vi "ACQ get internal temp.vi"(4 "pomiar temp (T)":bool=TRUE, 6 "i":i32, 7 "Urządzenie":tag, 8 "error in (no error)":errorcluster, 9 "div (300)":i32=300, 11 "Tasks ref in":T1) -> (0 "error out":errorcluster, 3 "Tasks ref out":T1, 5 "DevTemp":dbl)   [LabVIEW 2014]
doc: "Odczytuje temperaturę urządzenia co zadaną liczbę iteracji (div)\nprzerywając zadania pomiarowe.\n(div 125 to ok 1 sek przy pętli ok 0,008s)"
uses:
  Kontrolki/KartaDAQ/ACQ all read tasks.ctl
  <resource>/objmgr/daqmx.rc
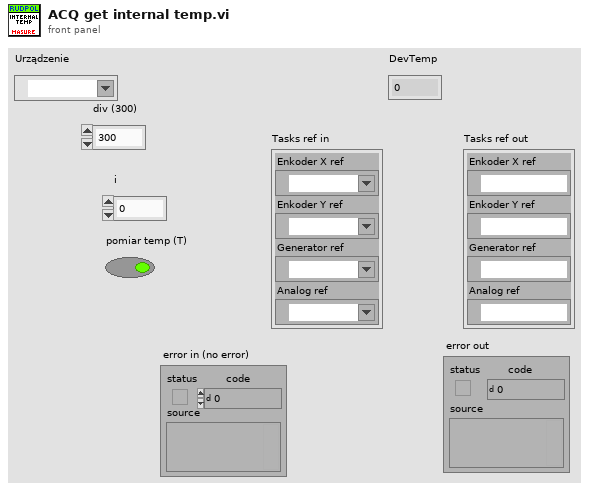
[diagram p1: front panel]
types:
  T1 = typedef "ACQ all read tasks.ctl" = cluster{"Analog ref":refnum<k21>, "Enkoder X ref":refnum<k21>, "Enkoder Y ref":refnum<k21>, "Generator ref":refnum<k21>}
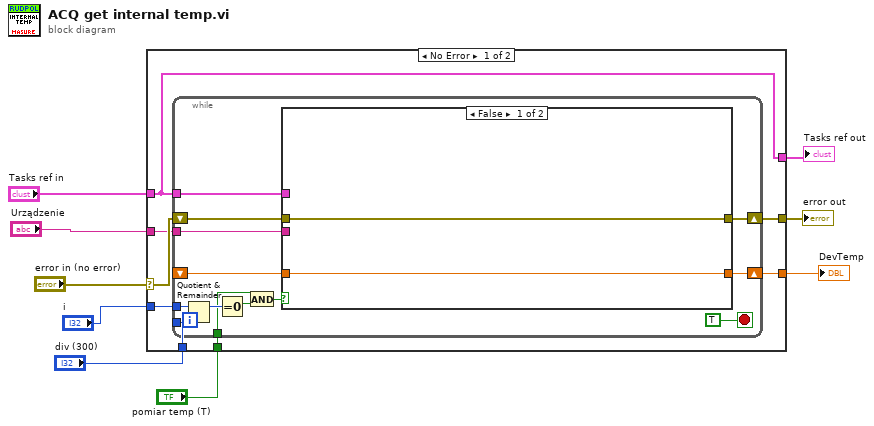
[diagram p0: block diagram]
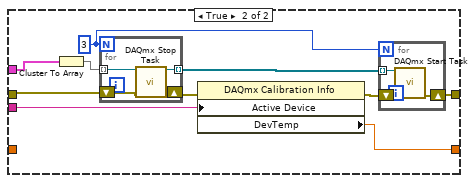
[diagram p2: hidden frame]
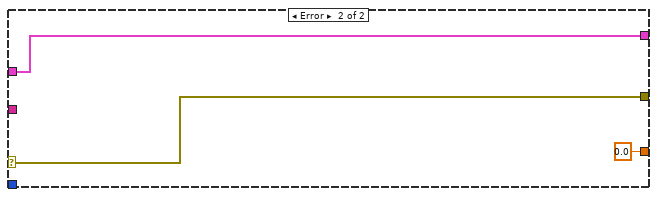
[diagram p3: hidden frame]
diagram:
  n1 = case shown="No Error" "error in (no error)" {
    selector: "error in (no error)" -> [w17 w52]
    tunnel: [w15 w52] -> w8
    tunnel: "Tasks ref in" -> [w16 w51]
    tunnel: [w16 w51] -> w6
    tunnel: "Urządzenie" -> [w14 _]
    tunnel: "i" -> [w13 _]
    tunnel: "div (300)" -> [w12 _]
    tunnel: [w11 0.0 ("DevTemp")] -> w2
    tunnel: "pomiar temp (T)" -> [w10 _]
    frame No Error {
      n2 = while {
        tunnel: w16 -> [w29]
        tunnel: w14 -> [w27]
        tunnel: w13 -> [w25]
        tunnel: w12 -> [w24]
        shift-right: [w28] -> w15
        shift-left: w17 -> [w30]
        shift-right: [w23] -> w11
        shift-left: _ -> [w21]
        tunnel: w10 -> [w18]
        stop <- TRUE stop-if-true
        n3 = Quotient & Remainder(x=w25, y=w24) -> (x-y*floor(x/y)=w26:i32)  [unwired: 1 out]
        n4 = Equal To 0?(x=w26) -> (x = 0?=w19:bool)
        n5 = And(x=w18, y=w19) -> (x .and. y?=w20:bool)
        n6 = case shown="False" w20 {
          tunnel: w30 -> [w32 w37]
          tunnel: w29 -> [_ w36]
          tunnel: [w32 w40] -> w28
          tunnel: w27 -> [_ w38]
          tunnel: [w31 w33] -> w23
          tunnel: w21 -> [w31 _]
          frame False {
          }
          frame True {
            w34 = 3
            n7 = Cluster To Array(cluster=w36) -> (array=w35:refnum<k21>[])
            n8 = for {
              N: w34 -> [_]
              tunnel: [w49] -> w42 mode=indexing
              shift-right: [w48] -> w41
              shift-left: w37 -> [w47]
              tunnel: w35 -> [w46] mode=indexing
              n9 = call <vilib>:"DAQmx Stop Task.vi"("task/channels in"=w46, "error in"=w47) -> ("task out"=w49:refnum<k21>, "error out"=w48:errorcluster)  [unwired: 12 in]
            }
            n10 = property class="DAQmx Calibration Info"(error in=w41, "Active Device"=w38) -> (error out=w39:errorcluster, "DevTemp"=w33:dbl)  [unwired: 1 in, 1 out]
            n11 = for {
              N: w34 -> [_]
              tunnel: w42 -> [w45] mode=indexing
              shift-right: [w44] -> w40
              shift-left: w39 -> [w43]
              n12 = call <vilib>:"DAQmx Start Task.vi"("task/channels in"=w45, "error in"=w43) -> ("error out"=w44:errorcluster)  [unwired: 12 in, 1 out]
            }
          }
        }
      }
    }
    frame Error {
    }
  }
  "error out" <- w8
  "Tasks ref out" <- w6
  "DevTemp" <- w2
